vi "Create stock design request.vi"(8 "error in":errorcluster, 9 "Stock Design Index":i32, 10 "Method Name":string, 11 "Mathcad version":i32) -> (0 "error out":errorcluster, 2 "DesignRequest":T1, 3 "Request File Name":string)   [LabVIEW 2012]
uses:
  Design Request.ctl
  Variable cluster.ctl
  Design Server.lvlib
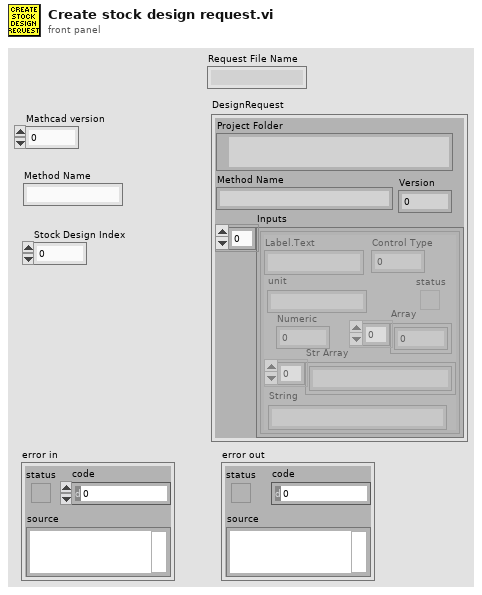
[diagram p1: front panel]
types:
  T1 = typedef "Design Server.lvlib/Design Request.ctl" = cluster{"Project Folder":path, "Method Name":string, "Inputs":T2, "Version":i32}
  T2 = typedef "Design Server.lvlib/Variable cluster.ctl" = cluster{"Label.Text":string, "Control Type":u32, "Numeric":dbl, "Array":dbl[], "status":bool, "Str Array":string[], "String":string, "unit":string}[]
  T3 = typedef "Method.ctl" = cluster{"Title":string, "About":string, "Input Parameters":cluster{"Description":string, "Name":string, "Min":string, "Max":string, "Default":string, "Units":string, "Increment":string, "Stock designs":string[]}[], "AutoCAD drawings":cluster{"File Name":string, "AC Variables":string[]}[], "Stock file names":string[], "Publish files":string[], "Display images":string[]}
  T4 = cluster{"Description":string, "Name":string, "Min":string, "Max":string, "Default":string, "Units":string, "Increment":string, "Stock designs":string[]}[]
  T5 = cluster{"Label.Text":string, "Control Type":u32, "Numeric":dbl, "Array":dbl[], "status":bool, "Str Array":string[], "String":string, "unit":string}
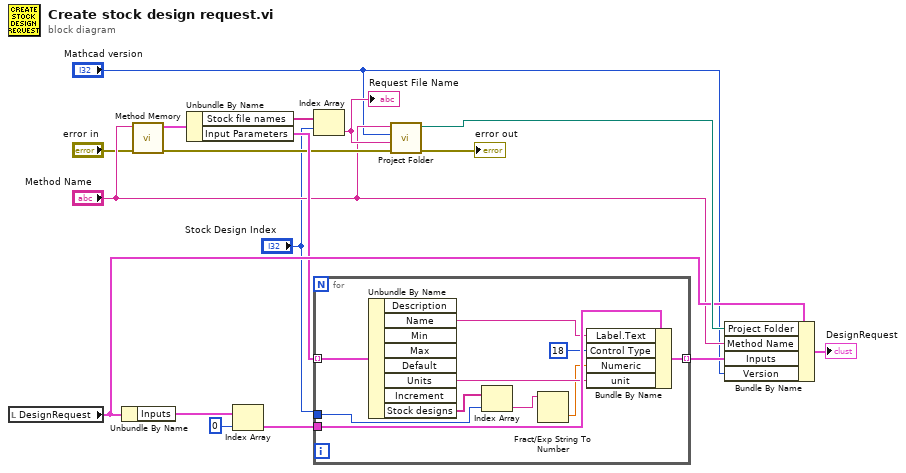
[diagram p0: block diagram]
diagram:
  n1 = local read "DesignRequest"() -> (w14:T1)
  n2 = Unbundle By Name(w14) -> ("Inputs"=w12:T2)
  n3 = call "Method Memory.vi"("error in"="error in", "Method Name"="Method Name") -> ("error out"=w6:errorcluster, "Method Out"=w15:T3)  [unwired: 7 in, 1 out]
  n4 = Unbundle By Name(w15) -> ("Stock file names"=w8:string[], "Input Parameters"=w13:T4)
  n5 = Index Array(array=w12, index=0) -> (element=w10:T5)
  n6 = Index Array(array=w8, index="Stock Design Index") -> (element=w7:string)
  "Request File Name" <- w7
  n7 = for {
    tunnel: w13 -> [w27] mode=indexing
    tunnel: "Stock Design Index" -> [w25]
    tunnel: w10 -> [w24]
    tunnel: [w23] -> w11 mode=indexing
    n8 = Unbundle By Name(w27) -> ("Name"=w22:string, "Units"=w21:string, "Stock designs"=w26:string[])  [unwired: 5 out]
    n9 = Index Array(array=w26, index=w25) -> (element=w20:string)
    n10 = Fract/Exp String To Number(string=w20) -> (number=w19:dbl)  [unwired: 3 in, 1 out]
    n11 = Bundle By Name(cluster=w24, "Label.Text"=w22, "Control Type"=u32 18, "Numeric"=w19, "unit"=w21) -> (w23:T5)
  }
  n12 = call "Project Folder.vi"("error in (no error)"=w6, "Request File Name"=w7, "Revision"="Mathcad version", "Method"="Method Name") -> ("error out"=→"error out":errorcluster, "Completed Design path"=w16:path)  [unwired: 6 in]
  n13 = Bundle By Name(cluster=w14, "Project Folder"=w16, "Method Name"="Method Name", "Inputs"=w11, "Version"="Mathcad version") -> (→"DesignRequest":T1)
